vi "Lookup Base Protection Class.vi"(8 "error in (no error)":errorcluster, 10 "Protection in":string, 11 "Class Lookup":variant) -> (0 "error out":errorcluster, 2 "Protection.lvclass":refnum<class "Protection.lvclass">, 3 "Class Lookup out":variant)   [LabVIEW 2018, in "Instrument Addon Shared.lvlib"]
uses:
  Instrument Addon Shared.lvlib
  Source/Addon/Support Libraries/Protections.lvlibp/Parent Protection/Protection.lvclass
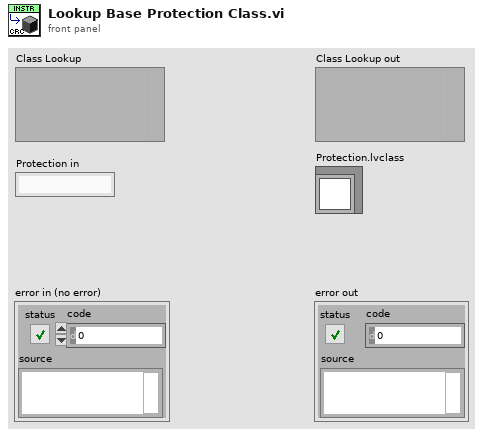
[diagram p1: front panel]
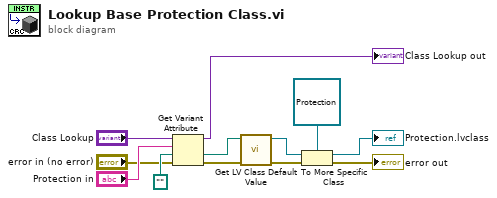
[diagram p0: block diagram]
diagram:
  n1 = Get Variant Attribute(Variant="Class Lookup", name="Protection in", default value (empty Variant)=path "", error in="error in (no error)") -> (duplicate Variant=→"Class Lookup out":variant, value=w7:path, error out=w8:errorcluster)  [unwired: 1 out]
  n2 = call <vilib>:"Get LV Class Default Value.vi"("error in (no error)"=w8, "class path"=w7) -> ("error out"=w9:errorcluster, "object"=w11:refnum<class>)  [unwired: 8 in]
  n3 = To More Specific Class(target class=refnum<class "Protection.lvclass"> refnum ("Protections.lvlibp:Protection.lvclass"), reference=w11, error in=w9) -> (specific class reference=→"Protection.lvclass":refnum<class "Protection.lvclass">, error out=→"error out":errorcluster)
